vi "Explore to Path.vi"(8 "error in (no error)":errorcluster, 10 "Select Directory? (F: Open Directory)":bool, 11 "Path":path) -> (0 "error out":errorcluster)   [LabVIEW 2017, in "csm-ui-support.lvlib"]
uses:
  csm-ui-support.lvlib
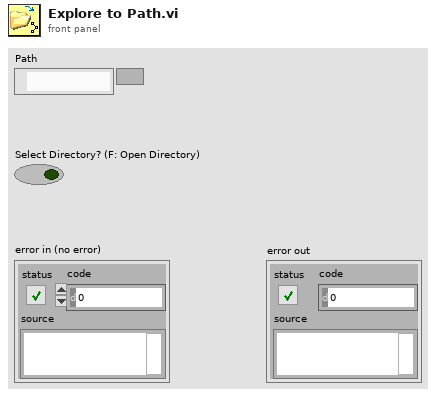
[diagram p1: front panel]
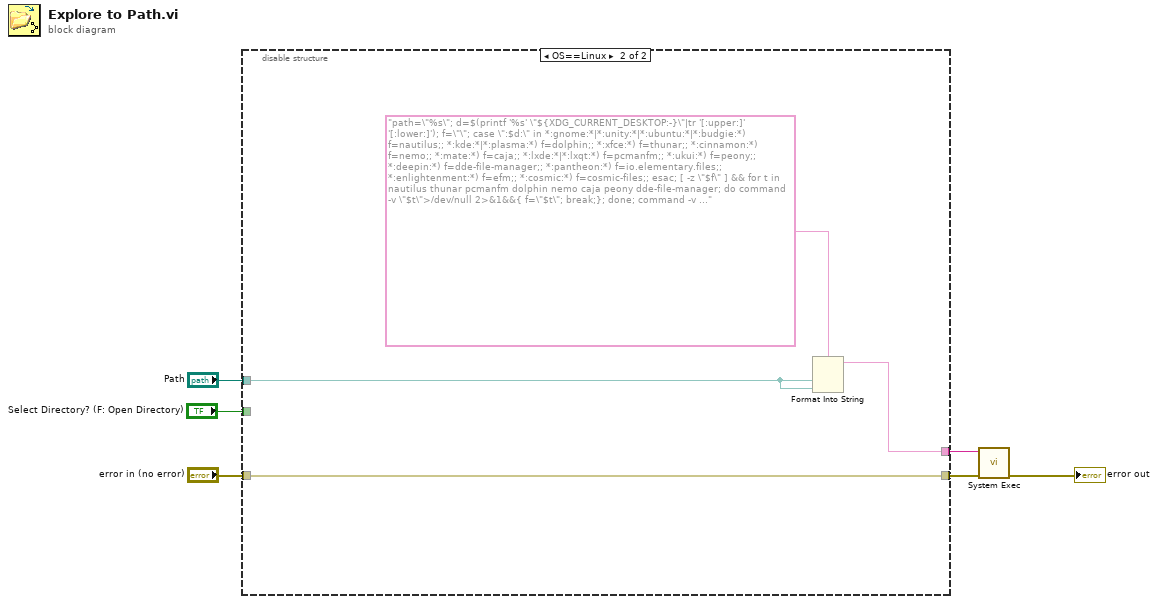
[diagram p0: block diagram]
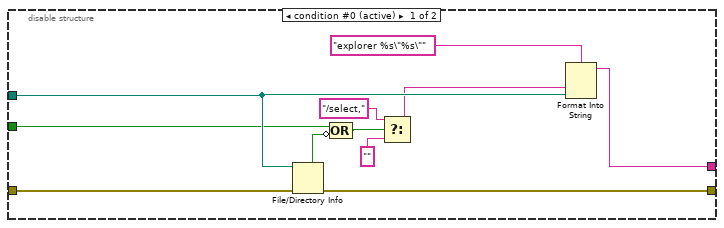
[diagram p2: hidden frame]
diagram:
  n1 = disable-structure shown="OS==Linux" {
    disable-tunnel: "Path" -> [w17 w19]
    disable-tunnel: [w12 w21] -> w4
    disable-tunnel: [w10 w18] -> w3
    disable-tunnel: "error in (no error)" -> [w8 w21]
    disable-tunnel: "Select Directory? (F: Open Directory)" -> [w7 _]
    frame condition #0 (active) {
      n2 = File/Directory Info(path=w17, error in=w8) -> (directory=w11:bool, error out=w12:errorcluster)  [unwired: 5 out]
      n3 = Compound Arithmetic op=OR(w7, invert w11) -> (w13:bool)
      n4 = Select(t="/select," ("format string"), s=w13, f="") -> (s? t:f=w14:string)
      n5 = Format Into String(format string="explorer %s\"%s\"", w14, w17) -> (resulting string=w10:string)  [unwired: 2 in, 1 out]
    }
    frame condition #1 {
      n6 = Format Into String(format string="path=\"%s\"; d=$(printf '%s' \"${XDG_CURRENT_DESKTOP:-}\"|tr '[:upper:]' '[:lower:]'); f=\"\"; case \":$d:\" in *:gnome:*|*:unity:*|*:ubuntu:*|*:budgie:*) f=nautilus;; *:kde:*|*:plasma:*) f=dolphin;; *:xfce:*) f=thunar;; *:cinnamon:*) f=nemo;; *:mate:*) f=caja;; *:lxde:*|*:lxqt:*) f=pcmanfm;; *:ukui:*) f=peony;; *:deepin:*) f=dde-file-manager;; *:pantheon:*) f=io.elementary.files;; *:enlightenment:*) f=efm;; *:cosmic:*) f=cosmic-files;; esac; [ -z \"$f\" ] && for t in nautilus thunar pcmanfm dolphin nemo caja peony dde-file-manager; do command -v \"$t\">/dev/null 2>&1&&{ f=\"$t\"; break;}; done; command -v \"$f\">/dev/null 2>&1||f=xdg-open; [ \"$f\" = nautilus ] && nautilus --no-desktop \"$path\" 2>/dev/null||\"$f\" \"$path\"", w19, w19) -> (resulting string=w18:string)  [unwired: 2 in, 1 out]
    }
  }
  n7 = call <vilib>:"System Exec.vi"("error in (no error)"=w4, "command line"=w3) -> ("error out"=→"error out":errorcluster)  [unwired: 6 in, 3 out]
